vi "Stop Core.vi"(10 "final error code":i32, 11 "Measure Object in":refnum<class "Measure Object.lvclass">) -> (3 "Measure Object out":refnum<class "Measure Object.lvclass">)   [LabVIEW 2015, in "Measure Object.lvclass"]
doc: "(<B>Filename</B>: Actor Framework.lvlib:Actor.lvclass:Stop Core.vi)\n\nDefines what the actor does before it stops. Use the <B>final error code</B> input to determine whether the actor shut down in response to an error.\n\nBy default, this method does nothing. A descendant class may override it to define behavior, such as shutting down any processes the actor initiated in its override of the Actor Core method."
uses:
  Measure Object.lvclass
  Measure Object.lvclass/Measure Object.ctl
  <vilib>/ActorFramework/Actor/Actor.lvclass
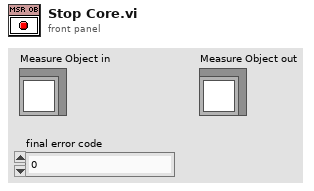
[diagram p1: front panel]
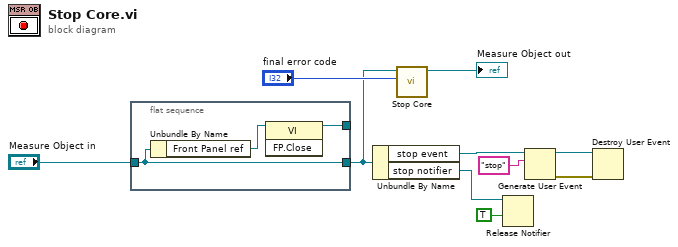
[diagram p0: block diagram]
diagram:
  n1 = flat-sequence {
    tunnel: "Measure Object in" -> [w13]
    tunnel: [w13] -> w1
    tunnel: [w11] -> _
    frame #0 {
      n2 = Unbundle By Name(w13) -> ("Front Panel ref"=w12:refnum<vi>)
      n3 = invoke class="VI" method="FP.Close"(reference=w12) -> (reference out=w11:refnum<vi>)  [unwired: 2 in, 2 out]
    }
  }
  n4 = Unbundle By Name(w1) -> ("stop event"=w4:refnum<user-event>, "stop notifier"=w3:refnum<notifier>)
  n5 = call-parent "Stop Core.vi"("final error code"="final error code", "Actor in"=w1) -> ("Actor out"=→"Measure Object out":refnum<class "Measure Object.lvclass">)  [unwired: 9 in]
  n6 = Release Notifier(notifier=w3, force destroy? (F)=TRUE) -> ()  [unwired: 1 in, 3 out]
  n7 = Generate User Event(user event=w4, event data cluster="stop" ("event data")) -> (user event out=w5:refnum<user-event>, error out=w6:errorcluster)  [unwired: 2 in]
  n8 = Destroy User Event(user event=w5, error in=w6) -> ()  [unwired: 1 out]
